vi "MoveRelate.vi"(8 "error in (no error)":errorcluster, 11 "DMC_1000B in":refnum<class "DMC_1000B.lvclass">) -> (0 "error out":errorcluster, 3 "DMC_1000B out":refnum<class "DMC_1000B.lvclass">)   [LabVIEW 2019, in "DMC_1000B.lvclass"]
uses:
  DMC_1000B.lvclass
  LLB/Commonly VI/Main Glb.vi
  LLB/DMC1000B/Dmc1000/Dmc1000.lvlib
  LLB/Commonly VI.lvlib
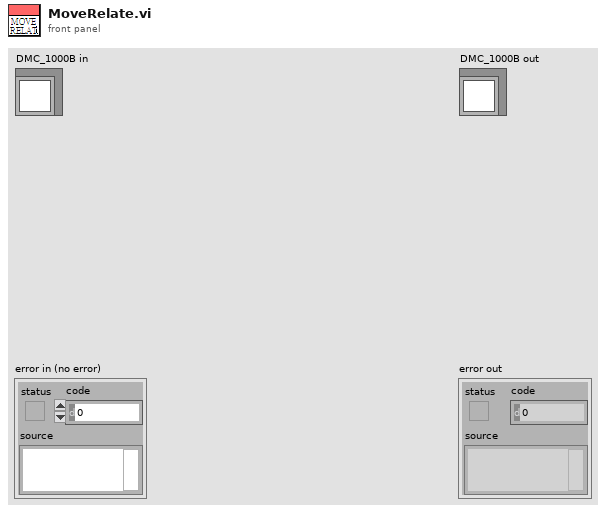
[diagram p1: front panel]
types:
  T1 = cluster{"AxisName":string, "Accel":dbl, "Deaccel":dbl, "Speed":dbl, "Sramp":dbl}[]
  T2 = cluster{"AxisName":string, "Accel":dbl, "Deaccel":dbl, "Speed":dbl, "Sramp":dbl}
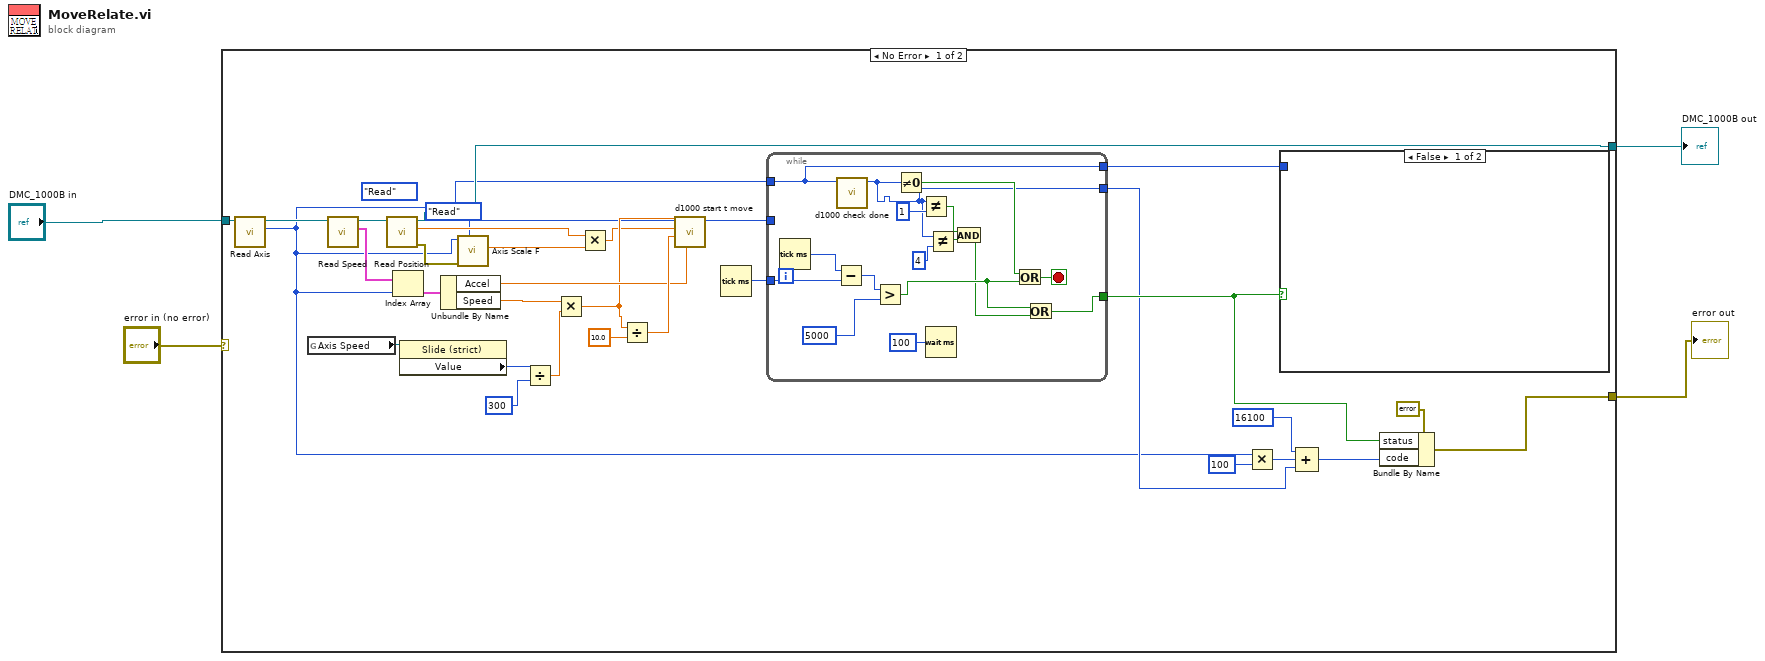
[diagram p0: block diagram]
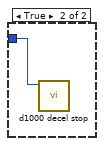
[diagram p2: hidden frame]
diagram:
  n1 = case shown="No Error" "error in (no error)" {
    selector: "error in (no error)" -> [_ w55]
    tunnel: "DMC_1000B in" -> [w11 w54]
    tunnel: [w9 w54] -> w2
    tunnel: [w10 w55] -> w1
    frame No Error {
      (unwired) enum16{"Initial", "Read"}."Read" ("Enum")
      n2 = call-dynamic "Read Axis.vi"("AxisCard in"=w11) -> ("Axis"=w5:u32, "AxisCard out"=w36:refnum<class "DMC_1000B.lvclass">)  [unwired: 8 in, 1 out]
      n3 = global read "Main Glb.vi" "Axis Speed"() -> (w19:refnum<vi>)
      n4 = call-dynamic "Read Speed.vi"("AxisCard in"=w36) -> ("AxisSpeed"=w35:T1, "AxisCard out"=w24:refnum<class "DMC_1000B.lvclass">)  [unwired: 8 in, 1 out]
      n5 = call-dynamic "Read Position.vi"("AxisCard in"=w24) -> ("error out"=w6:errorcluster, "Position"=w13:dbl, "AxisCard out"=w9:refnum<class "DMC_1000B.lvclass">)  [unwired: 8 in]
      n6 = Index Array(array=w35, index=w5) -> (element=w34:T2)
      n7 = property class="Slide (strict)"(reference=w19) -> ("Value"=w18:i32)  [unwired: 1 in, 2 out]
      n8 = Unbundle By Name(w34) -> ("Accel"=w21:dbl, "Speed"=w16:dbl)
      n9 = call "Axis Scale F.vi"("Enum"=enum16{"Initial", "Read"}."Read", "error In"=w6, "Axis"=w5) -> ("Scale"=w7:dbl)  [unwired: 7 in, 1 out]
      n10 = Divide(x=w18, y=300) -> (x/y=w15:dbl)
      n11 = Multiply(x=w16, y=w15) -> (x*y=w14:dbl)
      n12 = Multiply(x=w13, y=w7) -> (x*y=w12:dbl)
      n13 = Divide(x=w14, y=10.0) -> (x/y=w23:dbl)
      n14 = call "d1000 start t move.vi"("Tacc"=w21, "MaxVel"=w14, "StrVel"=w23, "Dist"=w12, "axis"=w5) -> ("function return"=w20:u32)  [unwired: 6 in]
      n15 = Tick Count (ms)() -> (millisecond timer value=w33:u32)
      n16 = while {
        tunnel: w5 -> [w47]
        tunnel: w33 -> [w51]
        tunnel: [w47] -> w32
        tunnel: [w45] -> w26
        tunnel: [w42] -> w25
        tunnel: w20 -> [_]
        stop <- w46 stop-if-true
        n17 = Tick Count (ms)() -> (millisecond timer value=w52:u32)
        n18 = Subtract(x=w52, y=w51) -> (x-y=w50:u32)
        n19 = call "d1000 check done.vi"("axis"=w47) -> ("function return"=w42:u32)  [unwired: 10 in]
        n20 = Greater?(x=w50, y=u32 5000) -> (0:w44:bool)
        n21 = Not Equal To 0?(x=w42) -> (x != 0?=w48:bool)
        n22 = Not Equal?(x=w42, y=u32 1) -> (x != y?=w39:bool)
        n23 = Wait (ms)(milliseconds to wait=u32 100) -> ()  [unwired: 1 out]
        n24 = Not Equal?(x=w42, y=u32 4) -> (x != y?=w40:bool)
        n25 = And(x=w39, y=w40) -> (x .and. y?=w38:bool)
        n26 = Or(x=w48, y=w44) -> (x .or. y?=w46:bool)
        n27 = Or(x=w44, y=w38) -> (x .or. y?=w45:bool)
      }
      n28 = Multiply(x=w5, y=u32 100) -> (x*y=w30:u32)
      n29 = case shown="False" w26 {
        tunnel: w32 -> [_ w37]
        frame False {
        }
        frame True {
          n30 = call "d1000 decel stop.vi"("axis"=w37) -> ()  [unwired: 10 in, 1 out]
        }
      }
      n31 = Compound Arithmetic op=ADD(16100, w30, w25) -> (w27:u32)
      n32 = Bundle By Name(cluster=errorcluster {"status"=FALSE, "code"=0, "source"=""} ("error constant"), "status"=w26, "code"=w27) -> (w10:errorcluster)
    }
    frame Error {
    }
  }
  "error out" <- w1
  "DMC_1000B out" <- w2
